vi "init.vi"(8 "error in (no error)":errorcluster, 10 "Resource":string, 11 "DmmNiPxi in":refnum<class "DmmNi.lvclass">) -> (0 "error out":errorcluster, 3 "DmmNiPxi out":refnum<class "DmmNi.lvclass">)   [LabVIEW 2023, in "DmmNi.lvclass"]
doc: "<b>Author:</b> Wolfgang\n<b>Description:</b> Method to initialize an instrument by resource name (defined in NI MAX) for any instrument category."
uses:
  DmmNi.lvclass
  DmmNi.lvclass/DmmNi.ctl
  Multimeter.lvclass
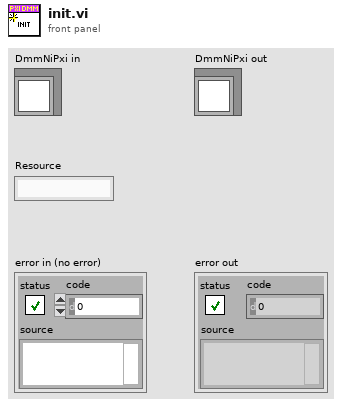
[diagram p1: front panel]
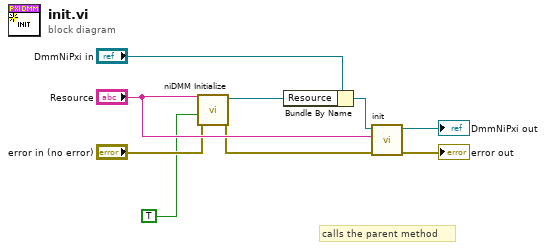
[diagram p0: block diagram]
diagram:
  # "calls the parent method"
  n1 = call <instrlib>:"niDMM Initialize.vi"("error in (no error)"="error in (no error)", "Reset"=TRUE, "Instrument Descriptor"="Resource") -> ("error out"=w3:errorcluster, "instrument handle out"=w2:refnum<k15>)  [unwired: 7 in]
  n2 = Bundle By Name(cluster="DmmNiPxi in", "Resource"=w2) -> (w5:refnum<class "DmmNi.lvclass">)
  n3 = call-parent "init.vi"("error in (no error)"=w3, "Resource"="Resource", "Instrument in"=w5) -> ("error out"=→"error out":errorcluster, "Instrument out"=→"DmmNiPxi out":refnum<class "DmmNi.lvclass">)  [unwired: 7 in]
